vi "SetROI.vi"(1 "RowBIn":i32=1, 2 "FirstCol":i32=1, 3 "ColBin":i32=1, 4 "LastRow":i32=512, 5 "FirstRow":i32=1, 6 "LastCol":i32=512) -> (0 "Error":bool)   [LabVIEW 2014]
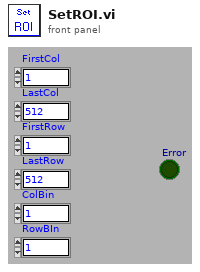
[diagram p1: front panel]
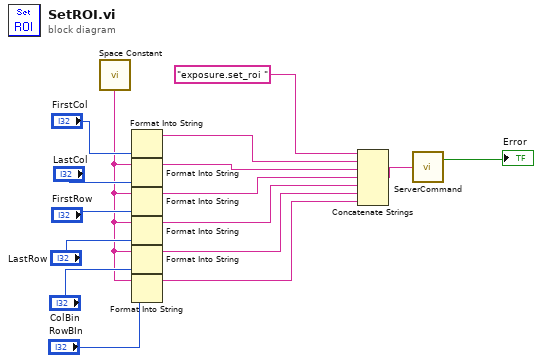
[diagram p0: block diagram]
diagram:
  n1 = call <vilib>:"Space Constant.vi"() -> ("String"=w1:string)
  n2 = Format Into String("FirstCol") -> (resulting string=w8:string)  [unwired: 3 in, 1 out]
  n3 = Format Into String(initial string=w1, "LastCol") -> (resulting string=w7:string)  [unwired: 2 in, 1 out]
  n4 = Format Into String(initial string=w1, "FirstRow") -> (resulting string=w6:string)  [unwired: 2 in, 1 out]
  n5 = Format Into String(initial string=w1, "LastRow") -> (resulting string=w5:string)  [unwired: 2 in, 1 out]
  n6 = Format Into String(initial string=w1, "ColBin") -> (resulting string=w4:string)  [unwired: 2 in, 1 out]
  n7 = Format Into String(initial string=w1, "RowBIn") -> (resulting string=w3:string)  [unwired: 2 in, 1 out]
  n8 = Concatenate Strings("exposure.set_roi " ("string"), w8, w7, w6, w5, w4, w3) -> (w10:string)
  n9 = call "ServerCommand.vi"("Command"=w10) -> ("Error"=→"Error":bool)  [unwired: 1 out]
